vi "RSZVB Get Coherent Signal Phase.vi"(8 "error in (no error)":errorcluster {"code" format="%.0x"}, 9 "Port (1)":i32=1, 10 "Channel (1)":i32=1, 11 "VISA session":refnum<visa-resource-name>) -> (0 "error out":errorcluster {"code" format="%.0x"}, 1 "Phase":dbl format="%^.3e", 3 "dup VISA session":refnum<visa-resource-name>)   [LabVIEW 2011]
doc: "This VI returns the phase for the coherent signal at port no. <Pt> relative to the phase of the reference signal (SOURce<Ch>:CMODe:RPORt). \n\nNote(s):\n\n(1) This VI is not available for R&S ZVB instrument.\n\nRemote-control command(s):\nSOURce<Ch>:CMODe:PORT<Pt>:PHASe?"
uses:
  _utility/RSZVB Global Data.vi
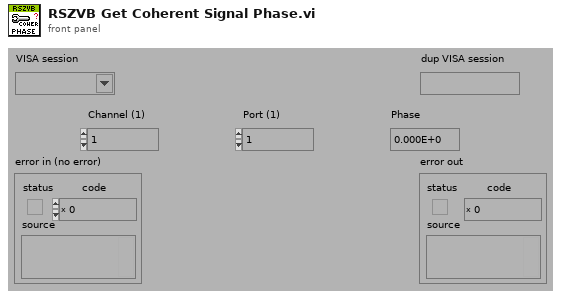
[diagram p1: front panel]
types:
  T1 = cluster{"Error Checking (T: On)":bool, "Installed Options":string[], "Data Valid?":bool, "Ports":i32, "Model":string[], "Option Checking (T: On)":bool}[]
  T2 = cluster{"Error Checking (T: On)":bool, "Installed Options":string[], "Data Valid?":bool, "Ports":i32, "Model":string[], "Option Checking (T: On)":bool}
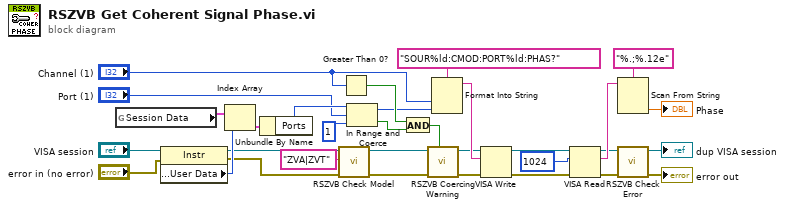
[diagram p0: block diagram]
diagram:
  n1 = global read "RSZVB Global Data.vi" "Session Data"() -> (w23:T1)
  n2 = property class="Instr"(reference="VISA session", error in="error in (no error)") -> (reference out=w2:refnum<visa-resource-name>, error out=w1:errorcluster, "General Settings:User Data"=w21:u32)
  n3 = Index Array(array=w23, index=w21) -> (element=w24:T2)
  n4 = Unbundle By Name(w24) -> ("Ports"=w20:i32)
  n5 = call "RSZVB Check Model.vi"("error in (no error)"=w1, "Model"="ZVA|ZVT", "VISA session"=w2) -> ("error out"=w3:errorcluster, "dup VISA session"=w4:refnum<visa-resource-name>)  [unwired: 7 in]
  n6 = Greater Than 0?(x="Channel (1)") -> (x > 0?=w30:bool)
  n7 = In Range and Coerce(upper limit=w20, x="Port (1)", lower limit=1) -> (coerced(x)=w19:i32, In Range?=w29:bool)
  n8 = And(x=w30, y=w29) -> (x .and. y?=w18:bool)
  n9 = call "RSZVB Coercing Warning.vi"("In Range?"=w18, "error in (no error)"=w3, "VISA session"=w4) -> ("error out"=w27:errorcluster, "dup VISA session"=w26:refnum<visa-resource-name>)  [unwired: 7 in]
  n10 = Format Into String(format string="SOUR%ld:CMOD:PORT%ld:PHAS?", "Channel (1)", w19) -> (resulting string=w28:string)  [unwired: 2 in, 1 out]
  n11 = VISA Write(VISA resource name=w26, write buffer=w28, error in (no error)=w27) -> (VISA resource name out=w14:refnum<visa-resource-name>, error out=w13:errorcluster)  [unwired: 1 out]
  n12 = VISA Read(VISA resource name=w14, byte count=u32 1024 ("byte count (0)"), error in (no error)=w13) -> (VISA resource name out=w16:refnum<visa-resource-name>, read buffer=w31:string, error out=w17:errorcluster)  [unwired: 1 out]
  n13 = Scan From String(format string="%.;%.12e", input string=w31) -> (output 1=→"Phase":dbl)  [unwired: 3 in, 3 out]
  n14 = call "RSZVB Check Error.vi"("error in (no error)"=w17, "VISA session"=w16) -> ("error out"=→"error out":errorcluster, "dup VISA session"=→"dup VISA session":refnum<visa-resource-name>)  [unwired: 8 in]
